vi "pythonstring.vi"(1 "Result Body":string) -> (0 "ETA":i32)   [LabVIEW 2023]
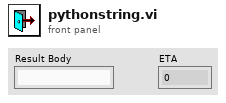
[diagram p1: front panel]
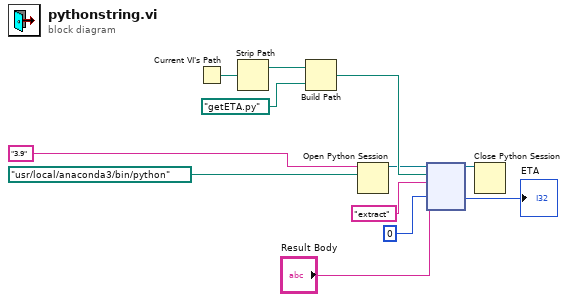
[diagram p0: block diagram]
diagram:
  n1 = Current VI's Path() -> (path=w5:path)
  n2 = Strip Path(path=w5) -> (stripped path=w4:path)  [unwired: 1 out]
  n3 = Build Path(base path=w4, name or relative path=path "getETA.py") -> (appended path=w7:path)
  n4 = Open Python Session(python version="3.9" ("Python version"), python path=path "/usr/local/anaconda3/bin/python" ("Python path")) -> (session out=w3:refnum<k35>)  [unwired: 1 in, 1 out]
  n5 = node(w3, w7, "extract" ("function name"), 0, "Result Body") -> (w8:refnum<k35>, →"ETA":i32)  [unwired: 2 in, 3 out]
  n6 = Close Python Session(session in=w8) -> ()  [unwired: 1 in, 1 out]
